vi "PC_NS_Signal init_communication.vi"(5 "# signal in NS ref":refnum<vi>, 7 "sig queue":refnum<queue>, 8 "error in (no error)":errorcluster, 11 "PC_NS_Signal in":refnum<class "PC_NS_Signal.lvclass">) -> (0 "error out":errorcluster, 3 "PC_NS_Signal out":refnum<class "PC_NS_Signal.lvclass">)   [LabVIEW 2018, in "PC_NS_Signal.lvclass"]
uses:
  PC_NS_Signal.lvclass
  PC_NS_Signal.lvclass/PC_NS_Signal.ctl
  <resource>/objmgr/ni.var.rc
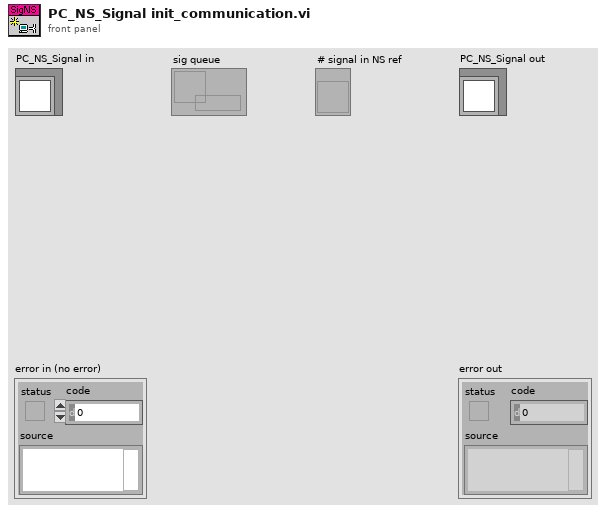
[diagram p1: front panel]
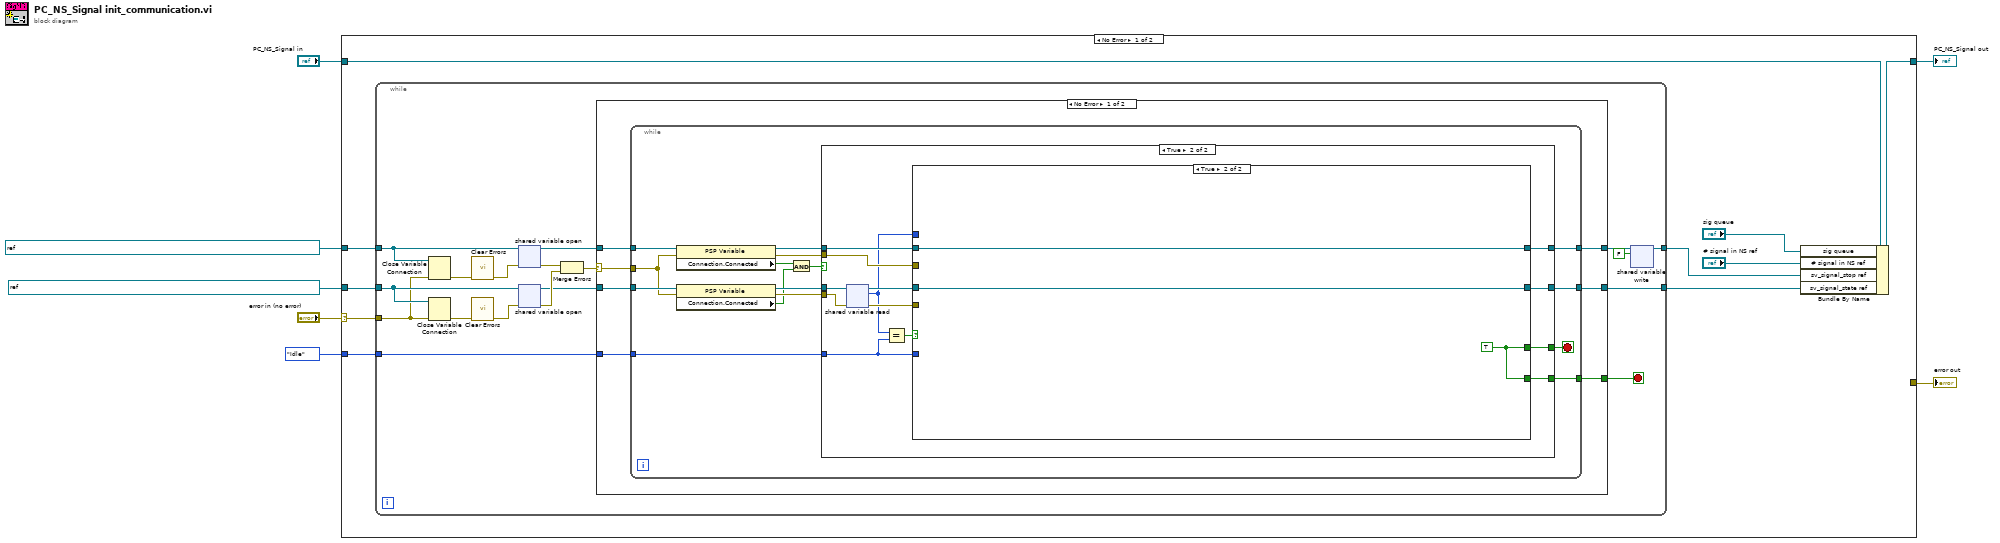
[diagram p0: block diagram]
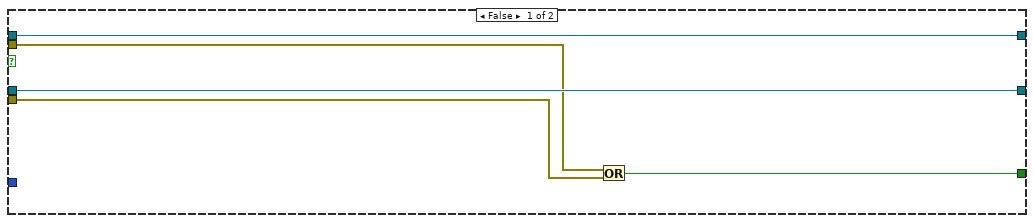
[diagram p2: hidden frame]
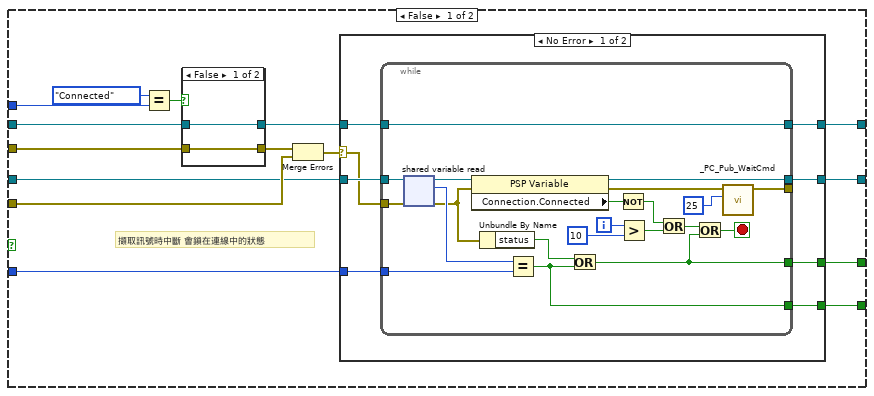
[diagram p3: hidden frame]
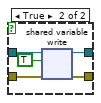
[diagram p4: hidden frame]
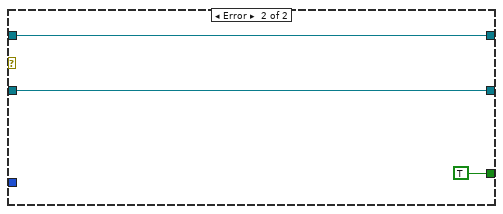
[diagram p5: hidden frame]
diagram:
  n1 = case shown="No Error" "error in (no error)" {
    selector: "error in (no error)" -> [w17 w136]
    tunnel: enum8{"Idle", "Init", "Connected", "Stop"}."Idle" ("y") -> [w16 _]
    tunnel: [_ w136] -> w6
    tunnel: [w14 w135] -> w5
    tunnel: "PC_NS_Signal in" -> [w15 w135]
    tunnel: refnum<k21> "ni.var.psp://NI-sbRIO/_RT_CtrlLoop_SigTrnsfr_Variable/Signal_Stop_Bool" ("shared variable refnum in") -> [w9 _]
    tunnel: refnum<k21> "ni.var.psp://NI-sbRIO/_RT_CtrlLoop_SigTrnsfr_Variable/Signal_RT_Status" ("shared variable refnum in") -> [w8 _]
    frame No Error {
      n2 = while {
        tunnel: w17 -> [w25]
        tunnel: w16 -> [w35]
        tunnel: [w19] -> w13
        tunnel: [w34] -> w12
        tunnel: w9 -> [w27]
        tunnel: w8 -> [w26]
        stop <- w21 stop-if-true
        n3 = Close Variable Connection(8:w25, 11:w27) -> (0:w29:errorcluster)
        n4 = Close Variable Connection(8:w25, 11:w26) -> (0:w31:errorcluster)
        n5 = call <vilib>:"Clear Errors.vi"("error in (no error)"=w29) -> ("error out"=w28:errorcluster)  [unwired: 5 in, 1 out]
        n6 = call <vilib>:"Clear Errors.vi"("error in (no error)"=w31) -> ("error out"=w30:errorcluster)  [unwired: 5 in, 1 out]
        n7 = shared-variable-open(w27, w28) -> (w23:refnum<k21>, w33:errorcluster)
        n8 = shared-variable-open(w26, w30) -> (w22:refnum<k21>, w32:errorcluster)
        n9 = Merge Errors(w33, w32) -> (w24:errorcluster)
        n10 = case shown="No Error" w24 {
          selector: w24 -> [w37 _]
          tunnel: w35 -> [w42 _]
          tunnel: w22 -> [w41 w133]
          tunnel: [w40 w134] -> w20
          tunnel: [w39 w133] -> w34
          tunnel: w23 -> [w38 w134]
          tunnel: [w36 _] -> w21
          frame No Error {
            n11 = while {
              tunnel: w41 -> [w57]
              tunnel: w38 -> [w56]
              tunnel: w42 -> [w54]
              tunnel: [w46] -> w40
              tunnel: [w45] -> w39
              tunnel: w37 -> [w44]
              tunnel: [w43] -> w36
              stop <- w47 stop-if-true
              n12 = property class="PSP Variable"(reference=w56, error in=w44) -> (reference out=w52:refnum<k21>, error out=w51:errorcluster, "Connection.Connected"=w50:bool)
              n13 = property class="PSP Variable"(reference=w57, error in=w44) -> (reference out=w55:refnum<k21>, error out=w53:errorcluster, "Connection.Connected"=w49:bool)
              n14 = And(x=w50, y=w49) -> (x .and. y?=w48:bool)
              n15 = case shown="True" w48 {
                tunnel: w55 -> [w61 w75]
                tunnel: w54 -> [_ w69]
                tunnel: w53 -> [w59 w73]
                tunnel: w52 -> [w62 w72]
                tunnel: w51 -> [w60 w71]
                tunnel: [w58 w68] -> w47
                tunnel: [w62 w67] -> w46
                tunnel: [w61 w66] -> w45
                tunnel: [_ w64] -> w43
                frame False {
                  n16 = Or(x=w60, y=w59) -> (x .or. y?=w58:bool)
                }
                frame True {
                  n17 = shared-variable-read(w75, w73) -> (w70:refnum<k21>, w65:errorcluster, w63:enum8{"Idle", "Init", "Connected", "Stop"})
                  n18 = Equal?(x=w63, y=w69) -> (x = y?=w74:bool)
                  n19 = case shown="True" w74 {
                    tunnel: w72 -> [w90 w132]
                    tunnel: w71 -> [w89 _]
                    tunnel: w70 -> [w76 w131]
                    tunnel: w69 -> [w82 _]
                    tunnel: [w85 w130] -> w68
                    tunnel: [w84 w132] -> w67
                    tunnel: [w83 w131] -> w66
                    tunnel: w65 -> [w77 _]
                    tunnel: [w81 w130] -> w64
                    tunnel: w63 -> [w80 _]
                    frame False {
                      # "擷取訊號時中斷 會鎖在連線中的狀態"
                      n20 = Equal?(x=enum8{"Idle", "Init", "Connected", "Stop"}."Connected", y=w80) -> (x = y?=w78:bool)
                      n21 = case shown="False" w78 {
                        tunnel: w90 -> [w92 w97]
                        tunnel: w89 -> [w91 w96]
                        tunnel: [w91 w95] -> w88
                        tunnel: [w92 w94] -> w86
                        frame False {
                        }
                        frame True {
                          n22 = shared-variable-write(w97, w96, TRUE ("data in")) -> (w94:refnum<k21>, w95:errorcluster)
                        }
                      }
                      n23 = Merge Errors(w88, w77) -> (w87:errorcluster)
                      n24 = case shown="No Error" w87 {
                        selector: w87 -> [w100 _]
                        tunnel: w86 -> [w105 w128]
                        tunnel: [w99 TRUE] -> w85
                        tunnel: [w104 w128] -> w84
                        tunnel: [w103 w127] -> w83
                        tunnel: w76 -> [w102 w127]
                        tunnel: w82 -> [w101 _]
                        tunnel: [w98 _] -> w81
                        frame No Error {
                          n25 = while {
                            tunnel: w102 -> [w126]
                            tunnel: w100 -> [w125]
                            tunnel: [w111] -> w99
                            tunnel: [w121] -> w104
                            tunnel: w105 -> [w121]
                            tunnel: [w120] -> w103
                            tunnel: w101 -> [w117]
                            tunnel: [w108] -> _
                            tunnel: [w106] -> w98
                            i -> [w119]
                            stop <- w110 stop-if-true
                            n26 = shared-variable-read(w126, w125) -> (w124:refnum<k21>, w116:errorcluster, w123:enum8{"Idle", "Init", "Connected", "Stop"})
                            n27 = property class="PSP Variable"(reference=w124, error in=w116) -> (reference out=w120:refnum<k21>, error out=w109:errorcluster, "Connection.Connected"=w122:bool)
                            n28 = Unbundle By Name(w116) -> ("status"=w115:bool)
                            n29 = Equal?(x=w123, y=w117) -> (x = y?=w106:bool)
                            n30 = Or(x=w115, y=w106) -> (x .or. y?=w111:bool)
                            n31 = Not(x=w122) -> (.not. x?=w114:bool)
                            n32 = Greater?(x=w119, y=10) -> (0:w113:bool)
                            n33 = Or(x=w114, y=w113) -> (x .or. y?=w112:bool)
                            n34 = Or(x=w112, y=w111) -> (x .or. y?=w110:bool)
                            n35 = call "_PC_Pub_WaitCmd.vi"("milliseconds to wait"=u32 25, "error in (no error)"=w109) -> ("error out"=w108:errorcluster)  [unwired: 9 in]
                          }
                        }
                        frame Error {
                        }
                      }
                    }
                    frame True {
                      w130 = TRUE ("Connection.Connected")
                    }
                  }
                }
              }
            }
          }
          frame Error {
          }
        }
        n36 = shared-variable-write(w20, FALSE ("data in")) -> (w19:refnum<k21>)  [unwired: 1 in, 1 out]
      }
      n37 = Bundle By Name(cluster=w15, "sig queue"="sig queue", "# signal in NS ref"="# signal in NS ref", "sv_signal_stop ref"=w13, "sv_signal_state ref"=w12) -> (w14:refnum<class "PC_NS_Signal.lvclass">)
    }
    frame Error {
    }
  }
  "error out" <- w6
  "PC_NS_Signal out" <- w5
